vi "1B Spoof Position Update.vi"(9 "Old Position":cluster{"X Position":dbl, "Y Position":dbl}, 10 "dt":dbl, 11 "Robot Velocity":cluster{"X Position":dbl, "Y Position":dbl}) -> (3 "New Position":cluster{"X Position":dbl, "Y Position":dbl})   [LabVIEW 2011]
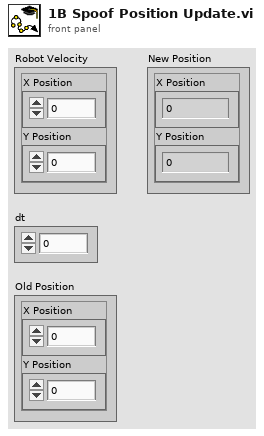
[diagram p1: front panel]
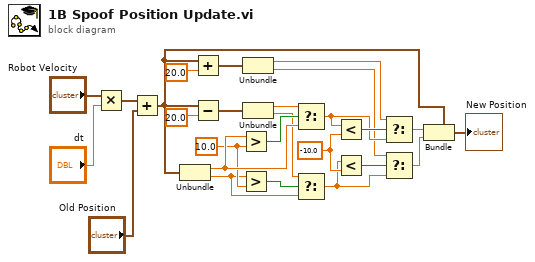
[diagram p0: block diagram]
diagram:
  w4 = -10.0 ("y")
  w9 = 10.0 ("y")
  n1 = Multiply(x="Robot Velocity", y="dt") -> (x*y=w25:cluster{"X Position":dbl, "Y Position":dbl})
  n2 = Add(x=w25, y="Old Position") -> (x+y=w18:cluster{"X Position":dbl, "Y Position":dbl})
  n3 = Unbundle(w18) -> ("X Position"=w15:dbl, "Y Position"=w7:dbl)
  n4 = Add(x=w18, y=20.0) -> (x+y=w16:cluster{"X Position":dbl, "Y Position":dbl})
  n5 = Subtract(x=w18, y=20.0) -> (x-y=w19:cluster{"X Position":dbl, "Y Position":dbl})
  n6 = Greater?(x=w15, y=w9) -> (0:w21:bool)
  n7 = Greater?(x=w7, y=w9) -> (0:w8:bool)
  n8 = Unbundle(w16) -> ("X Position"=w12:dbl, "Y Position"=w5:dbl)
  n9 = Unbundle(w19) -> ("X Position"=w14:dbl, "Y Position"=w6:dbl)
  n10 = Select(t=w14, s=w21, f=w15) -> (s? t:f=w11:dbl)
  n11 = Select(t=w6, s=w8, f=w7) -> (s? t:f=w3:dbl)
  n12 = Less?(x=w11, y=w4) -> (x < y?=w13:bool)
  n13 = Less?(x=w3, y=w4) -> (x < y?=w2:bool)
  n14 = Select(t=w12, s=w13, f=w11) -> (s? t:f=w10:dbl)
  n15 = Select(t=w5, s=w2, f=w3) -> (s? t:f=w1:dbl)
  n16 = Bundle(cluster=w18, "X Position"=w10, "Y Position"=w1) -> (→"New Position":cluster{"X Position":dbl, "Y Position":dbl})
